vi "Read File.vi"(8 "error in (no error)":errorcluster, 11 "[User] Cfg File in":refnum<class "[User] Cfg File.lvclass">) -> (0 "error out":errorcluster, 3 "[User] Cfg File out":refnum<class "[User] Cfg File.lvclass">)   [LabVIEW 2020, in "[User] Cfg File.lvclass"]
uses:
  [User] Cfg File.lvclass
  Control/config file.ctl
  [User] Cfg File.lvclass/[User] Cfg File.ctl
  <vilib>/Utility/config.llb/NI_LVConfig.lvlib
  <userlib>/_OpenG.lib/variantconfig/variantconfig.llb/openg_variant_configuration_file.lvlib
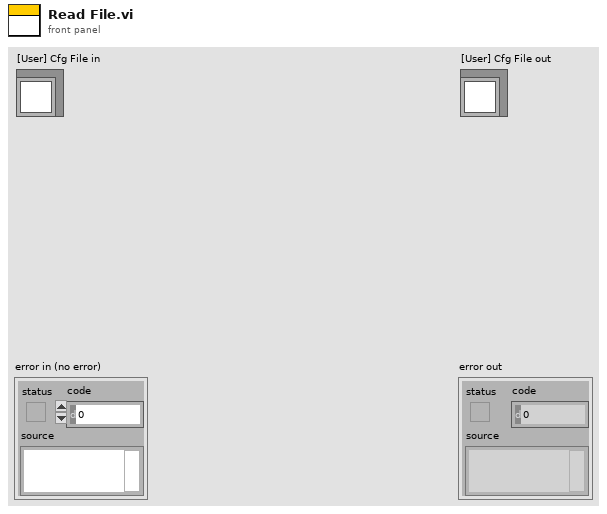
[diagram p1: front panel]
types:
  T1 = typedef "[User] Cfg File.lvclass/config file.ctl" = cluster{"login":cluster{"rmb_user":bool}}
  T2 = typedef "NI_LVConfig.lvlib/Config Data RefNum.ctl" = refnum<k1>
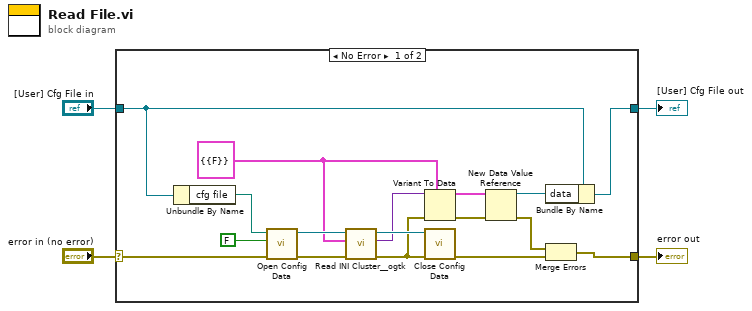
[diagram p0: block diagram]
diagram:
  n1 = case shown="No Error" "error in (no error)" {
    selector: "error in (no error)" -> [w21 w23]
    tunnel: [w12 w23] -> w3
    tunnel: [w10 w22] -> w1
    tunnel: "[User] Cfg File in" -> [w11 w22]
    frame No Error {
      w9 = T1 {"login"={"rmb_user"=FALSE}} ("config file")
      n2 = Unbundle By Name(w11) -> ("cfg file"=w20:path)
      n3 = call <vilib>:"Open Config Data.vi"("error in (no error)"=w21, "create file if necessary (T)"=FALSE, "configuration file path"=w20) -> ("error out"=w18:errorcluster, "refnum"=w17:T2)  [unwired: 6 in, 1 out]
      n4 = call <userlib>:"Read INI Cluster__ogtk.vi"("error in (no error)"=w18, "INI Fomatted Cluster Type"=w9, "refnum"=w17) -> ("error out"=w15:errorcluster, "INI Fomatted Cluster"=w14:variant, "dup refnum"=w16:T2)  [unwired: 4 in, 2 out]
      n5 = Variant To Data(error in=w15, type=w9, Variant=w14) -> (data=w7:T1, error out=w8:errorcluster)
      n6 = call <vilib>:"Close Config Data.vi"("error in (no error)"=w15, "refnum"=w16) -> ("error out"=w13:errorcluster)  [unwired: 8 in, 1 out]
      n7 = New Data Value Reference(data value=w7, error in=w8) -> (data value reference=w5:refnum<data-value>, error out=w6:errorcluster)
      n8 = Bundle By Name(cluster=w11, "data"=w5) -> (w10:refnum<class "[User] Cfg File.lvclass">)
      n9 = Merge Errors(w6, w13) -> (w12:errorcluster)
    }
    frame Error {
    }
  }
  "error out" <- w3
  "[User] Cfg File out" <- w1
